vi "Register Group Data Handler.vi"(8 "error in (no error)":errorcluster, 10 "Data Handler":refnum<class "SubscribedDataHandler.lvclass">, 11 "VolatusAPI in":refnum<class "VolatusAPI.lvclass">) -> (0 "error out":errorcluster, 3 "VolatusAPI out":refnum<class "VolatusAPI.lvclass">)   [LabVIEW 2020, in "Volatus.lvlib" / "VolatusAPI.lvclass"]
uses:
  VolatusAPI.lvclass
  lv-vecto/Vecto/SubscribedDataHandler/SubscribedDataHandler.lvclass
  VolatusAPI.lvclass/VolatusAPI.ctl
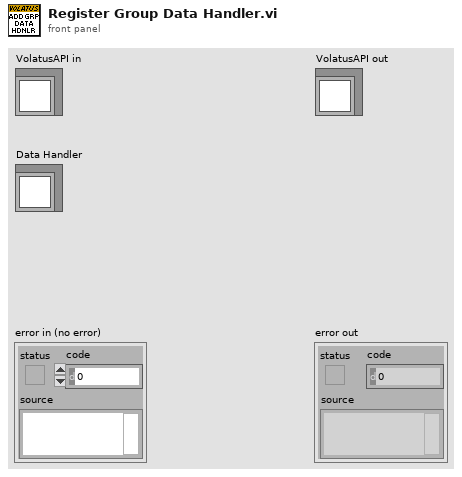
[diagram p1: front panel]
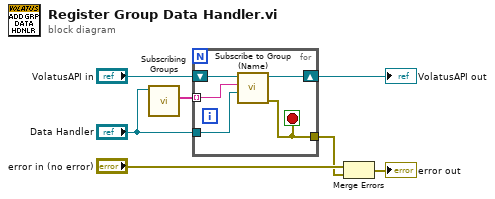
[diagram p0: block diagram]
diagram:
  n1 = call-dynamic "Subscribing Groups.vi"("SubscribedDataHandler in"="Data Handler") -> ("Subscribing Groups"=w7:string[])  [unwired: 9 in, 1 out]
  n2 = for {
    tunnel: w7 -> [w10] mode=indexing
    shift-right: [w9] -> w2
    shift-left: "VolatusAPI in" -> [w11]
    tunnel: [w12] -> w3
    tunnel: "Data Handler" -> [w8]
    stop <- w12 stop-if-true
    n3 = call "Subscribe to Group (Name).vi"("DataHandler (None)"=w8, "Group Name"=w10, "VolatusAPI in"=w11) -> ("error out"=w12:errorcluster, "VolatusAPI out"=w9:refnum<class "VolatusAPI.lvclass">)  [unwired: 6 in, 1 out]
  }
  "VolatusAPI out" <- w2
  n4 = Merge Errors("error in (no error)", w3) -> (→"error out":errorcluster)
